vi "Open DB.vi"(8 "error in (no error)":errorcluster, 9 "connection timeout (1)":i32=1, 10 "Connected String":string, 11 "SQLite_API in":refnum<class "SQLite_API.lvclass">) -> (0 "error out":errorcluster, 3 "SQLite_API out":refnum<class "SQLite_API.lvclass">)   [LabVIEW 2021, in "SQLite_API.lvclass"]
uses:
  <userlib>/John_Lib/DataBase/SQLite_API/SQLite_API.lvclass
  <userlib>/John_Lib/DataBase/SQLite_API/SQLite_API.lvclass/SQLite_API.ctl
  <vilib>/drjdpowell/SQLite Library/SQL Connection/Connection.lvclass
  <vilib>/drjdpowell/SQLite Library/SQL Connection/Open (string).vi
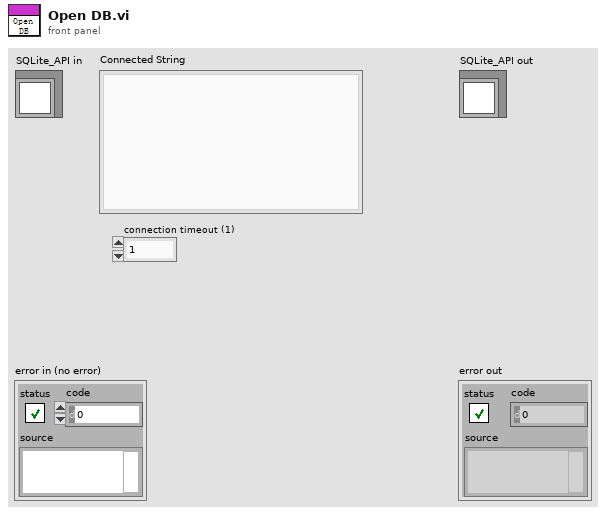
[diagram p1: front panel]
types:
  T1 = enum16{"New or existing", "Existing", "Read only"}
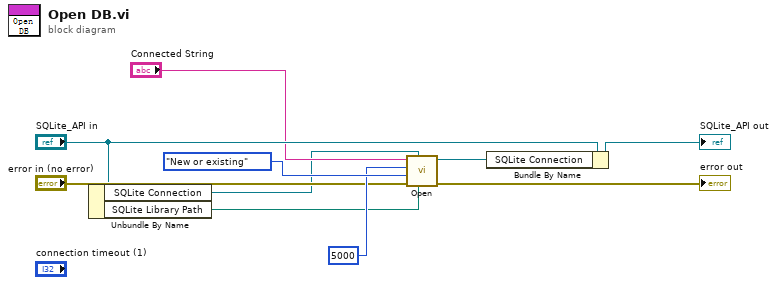
[diagram p0: block diagram]
diagram:
  n1 = Unbundle By Name("SQLite_API in") -> ("SQLite Connection"=w1:refnum<class "Connection.lvclass">, "SQLite Library Path"=w3:path)
  n2 = call-poly <vilib>:"Open.vi"("SQLite Library Path"=w3, "SQLite Connection type"=w1, "error in (no error)"="error in (no error)", "File Option"=T1."New or existing", "busy timeout (ms)"=5000, "db file"="Connected String") -> ("error out"=→"error out":errorcluster, "SQLite Connection"=w7:refnum<class "Connection.lvclass">)  [unwired: 4 in]
  n3 = Bundle By Name(cluster="SQLite_API in", "SQLite Connection"=w7) -> (→"SQLite_API out":refnum<class "SQLite_API.lvclass">)
